vi "Log Prefix Message.vi"(8 "error in (no error)":errorcluster, 10 "Log Prefix":string, 11 "Generic Controller in":refnum<class "Generic Plugin.lvclass">) -> (0 "error out":errorcluster, 2 "Log Prefix Message":T1, 3 "Generic Controller out":refnum<class "Generic Plugin.lvclass">)   [LabVIEW 2020, in "Generic Plugin.lvclass"]
uses:
  Generic Plugin.lvclass
  <userlib>/RxnRover/DynamicReentrant/src/Type Defs/Message.ctl
  <userlib>/RxnRover/DynamicReentrant/Dynamic Reentrant.lvlib
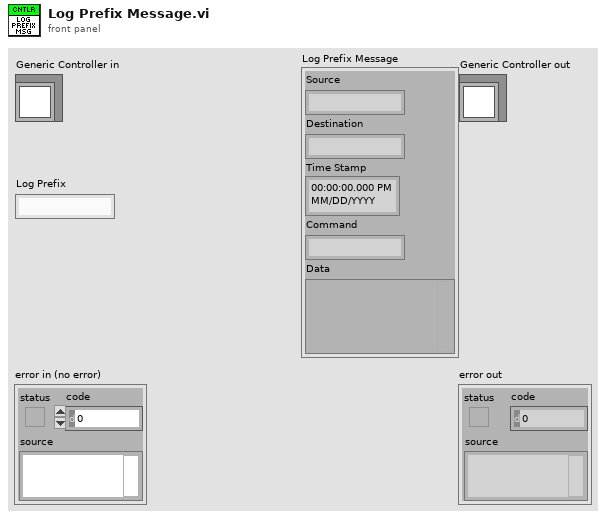
[diagram p1: front panel]
types:
  T1 = typedef "Dynamic Reentrant.lvlib/Message.ctl" = cluster{"Source":string, "Destination":string, "Time Stamp":timestamp, "Command":string, "Data":variant}
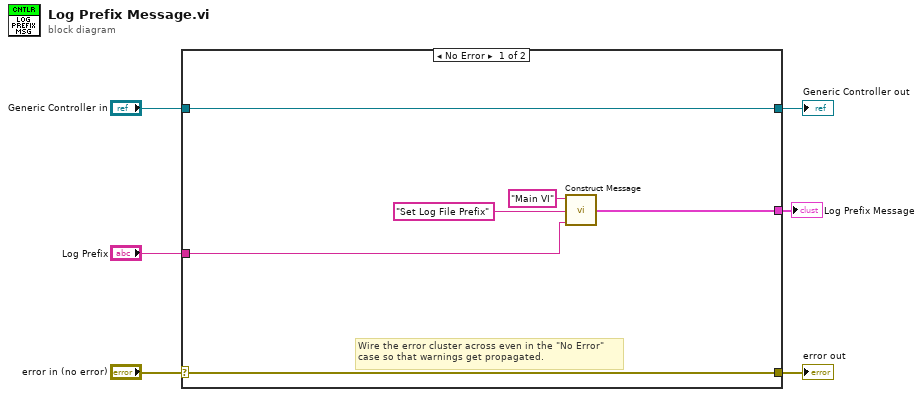
[diagram p0: block diagram]
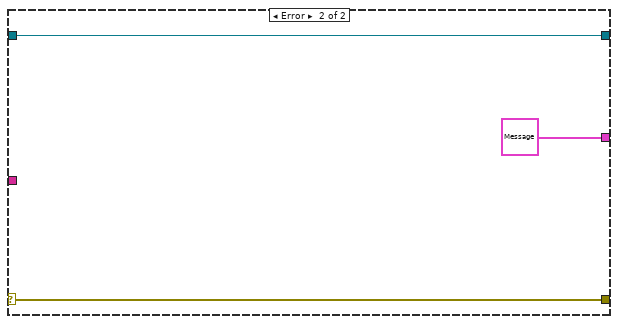
[diagram p2: hidden frame]
diagram:
  n1 = case shown="No Error" "error in (no error)" {
    selector: "error in (no error)" -> [w11 w15]
    tunnel: [w11 w15] -> w5
    tunnel: [w12 w14] -> w3
    tunnel: "Generic Controller in" -> [w12 w14]
    tunnel: [w7 T1 {"Source"="", "Destination"="", "Time Stamp"=timestamp(0 s since 1904-01-01), "Command"="", "Data"=variant} ("Message")] -> w2
    tunnel: "Log Prefix" -> [w8 _]
    frame No Error {
      # "Wire the error cluster across even in the \"No Error\"\ncase so that warnings get propagated."
      n2 = call <userlib>:"Construct Message.vi"("Data"=w8, "Command"="Set Log File Prefix", "Source"="Main VI") -> ("Message Cluster"=w7:T1)  [unwired: 3 in]
    }
    frame Error {
    }
  }
  "error out" <- w5
  "Generic Controller out" <- w3
  "Log Prefix Message" <- w2
